vi "StringFunctions.RemoveFileEnding.vi"(11 "FileString":string) -> (3 "FileName":string)   [LabVIEW 2016]
doc: "This VI reverses the given string, removes all letters up to the \".\" and reverses it again.\n\nAndreas Elmiger, 09.03.2017"
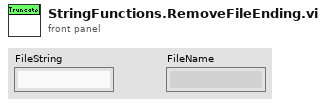
[diagram p1: front panel]
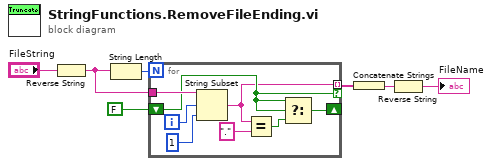
[diagram p0: block diagram]
diagram:
  n1 = Reverse String(1:"FileString") -> (0:w7:string)
  n2 = String Length(string=w7) -> (length=w6:i32)
  n3 = for {
    N: w6 -> [_]
    tunnel: w7 -> [w15]
    shift-right: [w11] -> _
    shift-left: FALSE -> [w12]
    tunnel: [w10] -> w4 mode=indexing if=w12
    i -> [w14]
    n4 = String Subset(string=w15, offset (0)=w14, length (rest)=1 ("length (rest)")) -> (substring=w10:string)
    n5 = Equal?(x=w10, y=".") -> (x = y?=w8:bool)
    n6 = Select(t=w12, s=w12, f=w8) -> (s? t:f=w11:bool)
  }
  n7 = Concatenate Strings(w4) -> (w3:string)
  n8 = Reverse String(1:w3) -> (0:→"FileName":string)
